vi "Wheel Ramping.vi"(0 "Joystick Value":dbl, 5 "Current Value":dbl, 7 "MaxRamping":dbl, 9 "MaxDeceleration":dbl) -> (4 "Changed Speed":dbl)   [LabVIEW 2020]
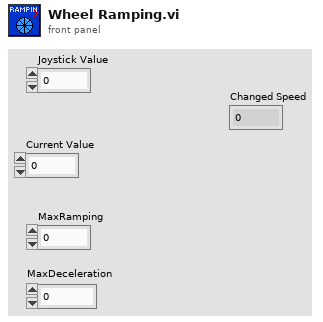
[diagram p1: front panel]
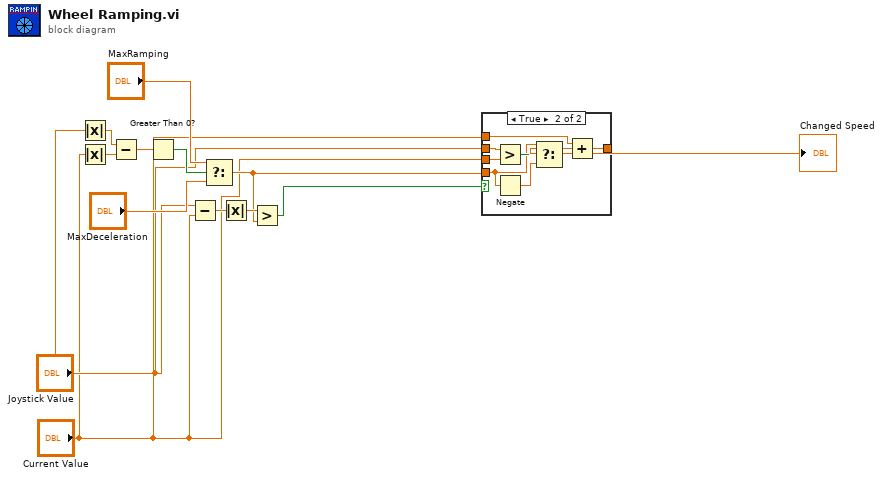
[diagram p0: block diagram]
diagram:
  n1 = Absolute Value(x="Joystick Value") -> (abs(x)=w13:dbl)
  n2 = Absolute Value(x="Current Value") -> (abs(x)=w12:dbl)
  n3 = Subtract(x=w13, y=w12) -> (x-y=w2:dbl)
  n4 = Greater Than 0?(x=w2) -> (x > 0?=w11:bool)
  n5 = Subtract(x="Joystick Value", y="Current Value") -> (x-y=w8:dbl)
  n6 = Select(t="MaxRamping", s=w11, f="MaxDeceleration") -> (s? t:f=w3:dbl)
  n7 = Absolute Value(x=w8) -> (abs(x)=w6:dbl)
  n8 = Greater?(x=w6, y=w3) -> (0:w7:bool)
  n9 = case shown="True" w7 {
    tunnel: [w14 w15] -> w5
    tunnel: "Joystick Value" -> [w14 w22]
    tunnel: "Current Value" -> [_ w21]
    tunnel: w3 -> [_ w19]
    tunnel: "Current Value" -> [_ w16]
    frame False {
    }
    frame True {
      n10 = Greater?(x=w22, y=w21) -> (0:w20:bool)
      n11 = Negate(x=w19) -> (-x=w18:dbl)
      n12 = Select(t=w19, s=w20, f=w18) -> (s? t:f=w17:dbl)
      n13 = Add(x=w16, y=w17) -> (x+y=w15:dbl)
    }
  }
  "Changed Speed" <- w5
